vi "Do Action.vi"(8 "error in (no error)":errorcluster, 9 "Display Queue":refnum<queue>, 10 "tlc_User Event Reference.ctl":T1, 11 "Play in":refnum<class "Play.lvclass">) -> (0 "error out":errorcluster)   [LabVIEW 2010, in "Play.lvclass"]
doc: "This instance of Do Action.vi is used to perform the functionality that was previously contained in the Play case of the consumer loop."
uses:
  Play.lvclass
  Controls/tlc_User Interface Command.ctl
  Controls/tlc_User Interface Data Type.ctl
  Controls/tlc_User Event Reference.ctl
  Play.lvclass/Play.ctl
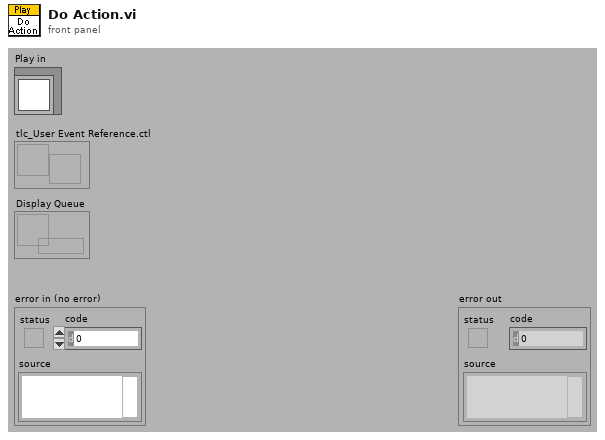
[diagram p1: front panel]
types:
  T1 = typedef "tlc_User Event Reference.ctl" = refnum<user-event>
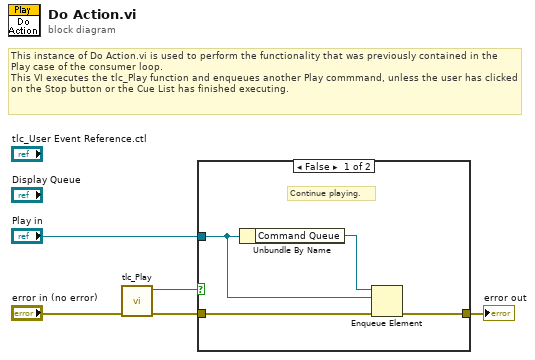
[diagram p0: block diagram]
diagram:
  # "This instance of Do Action.vi is used to perform the functionality that was previously contained in the Play case of the consumer loop.\nThis VI executes the tlc_Play function and enqueues another Play commmand, unless the user has clicked on the Stop button or the Cue List has finished executing."
  n1 = call "tlc_Play.vi"("error in (no error)"="error in (no error)") -> ("error out"=w2:errorcluster, "Stop?"=w4:bool)  [unwired: 9 in]
  n2 = case shown="False" w4 {
    tunnel: "Play in" -> [w8 _]
    tunnel: w2 -> [w7 w10]
    tunnel: [w6 w10] -> w1
    frame False {
      # "Continue playing."
      n3 = Unbundle By Name "Unbundle By Name"(w8) -> ("Command Queue"=w9:refnum<queue>)
      n4 = Enqueue Element(queue=w9, element=w8, error in (no error)=w7) -> (error out=w6:errorcluster)  [unwired: 1 in, 2 out]
    }
    frame True {
      # "Either the user clicked on the Stop button or the cue list has finished execution."
    }
  }
  "error out" <- w1
